vi "NI.Relays.vi"(6 "测试日志信息":refnum<queue>, 8 "error in":errorcluster caption="Error In", 9 "Relay.ON.OFF":bool caption="Relay.ON/OFF", 10 "Relay":T1(ring), 11 "DAQmx Device":tag) -> (0 "error out":errorcluster caption="Error Out")   [LabVIEW 2012, in "Lib_UEL.ATE.lvlib" / "Lib_PCI6221.lvlib"]
uses:
  Lib_PCI6221.lvlib
  <vilib>/DAQmx/write.llb/DAQmx Write (Digital Bool 1Line 1Point).vi
  <vilib>/DAQmx/create/channels.llb/DAQmx Create Channel (DO-Digital Output).vi
  <vilib>/DAQmx/miscellaneous.llb/DAQmx Fill In Error Info.vi
panel:
  # "V01 - Initial version. ~LiGuang 2011-05-12 \n V02 - 2013/1/11, 增加测试日志功能: 将测试信息加入到输入的队列中."
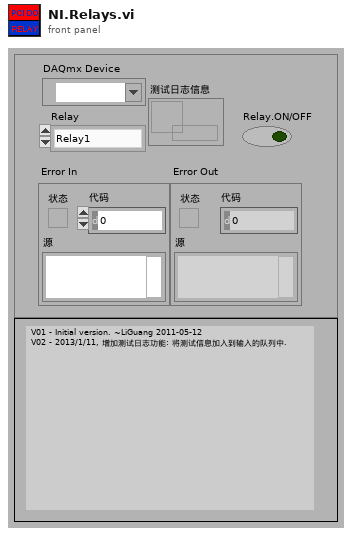
[diagram p1: front panel]
types:
  T1 = enum16{"Relay1", "Relay2", "Relay3", "Relay4", "Relay5", "Relay6", "Relay7", "Relay8", "Relay9", "Relay10"}
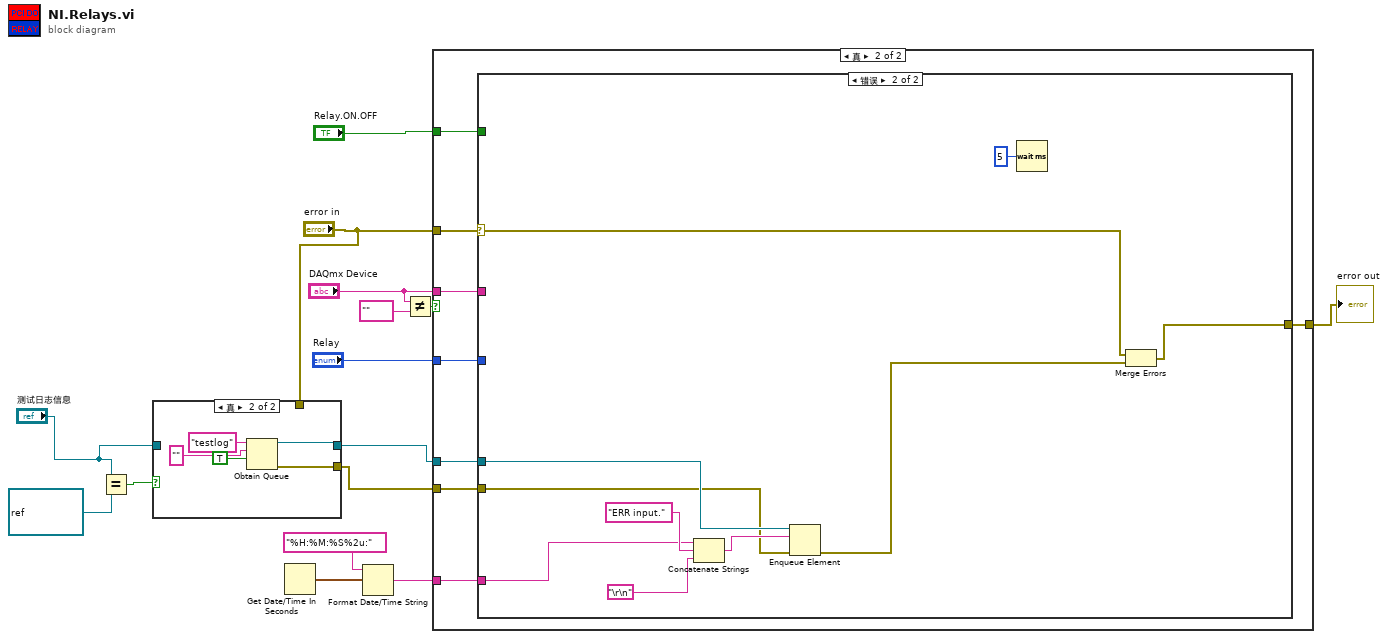
[diagram p0: block diagram]
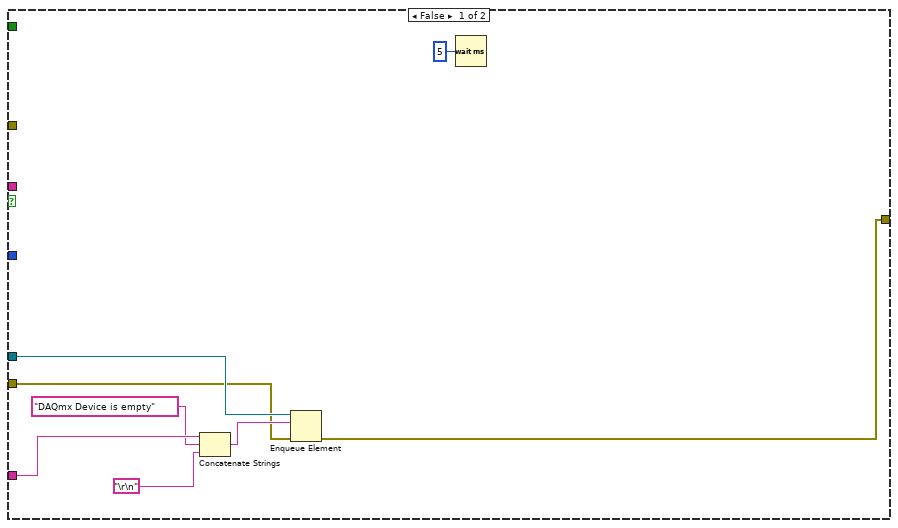
[diagram p3: hidden frame]
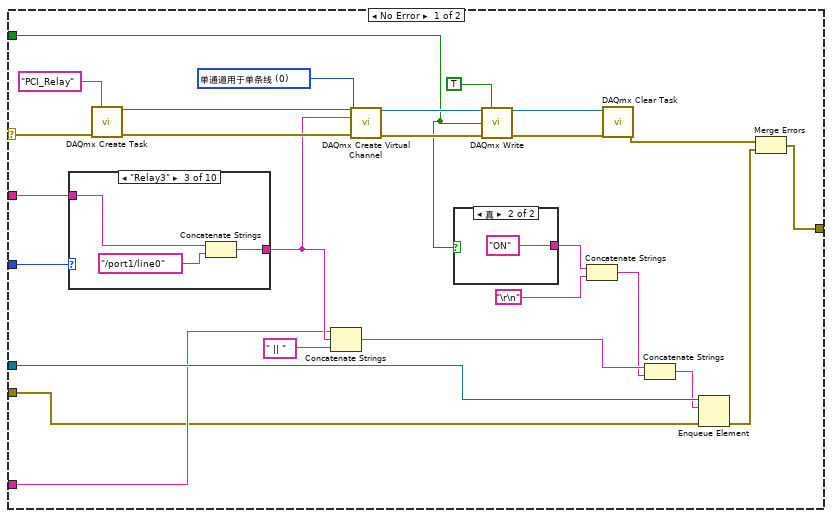
[diagram p4: hidden frame]
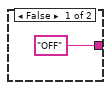
[diagram p5: hidden frame]
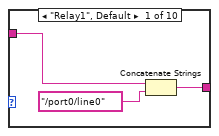
[diagram p6: hidden frame]
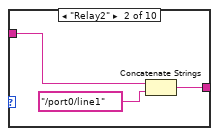
[diagram p7: hidden frame]
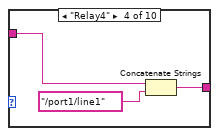
[diagram p8: hidden frame]
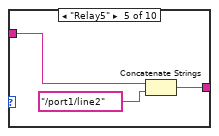
[diagram p9: hidden frame]
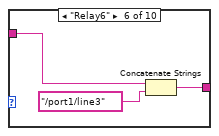
[diagram p10: hidden frame]
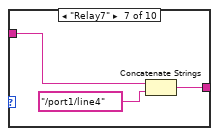
[diagram p11: hidden frame]
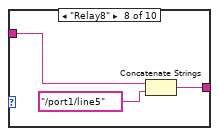
[diagram p12: hidden frame]
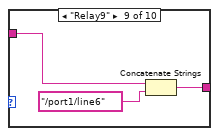
[diagram p13: hidden frame]
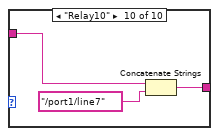
[diagram p14: hidden frame]
diagram:
  n1 = Equal?(x="测试日志信息", y=refnum<queue> refnum) -> (x = y?=w5:bool)
  n2 = case shown="真" w5 {
    tunnel: "测试日志信息" -> [w17 _]
    tunnel: [w17 w22] -> w3
    tunnel: [w16 w21] -> w1
    tunnel: "error in" -> [w16 _]
    frame False {
    }
    frame True {
      n3 = Obtain Queue(name (unnamed)="testlog" ("名称（未命名）"), element data type="" ("名称（未命名）"), create if not found? (T)=TRUE ("如未找到是否创建？(T)")) -> (queue out=w22:refnum<queue>, error out=w21:errorcluster)  [unwired: 2 in, 1 out]
    }
  }
  n4 = Get Date/Time In Seconds() -> (seconds since 1Jan1904=w8:timestamp)
  n5 = Format Date/Time String(time format string (%c)="%H:%M:%S%2u:" ("时间格式化字符串(%c)"), seconds (now)=w8) -> (date/time string=w7:string)  [unwired: 1 in]
  n6 = Not Equal?(x="DAQmx Device", y=tag "") -> (x != y?=w10:bool)
  n7 = case shown="真" w10 {
    tunnel: "error in" -> [_ w38]
    tunnel: [w25 w37] -> w15
    tunnel: "Relay" -> [_ w36]
    tunnel: "Relay.ON.OFF" -> [_ w35]
    tunnel: "DAQmx Device" -> [_ w34]
    tunnel: w3 -> [w30 w33]
    tunnel: w7 -> [w29 w32]
    tunnel: w1 -> [w23 w31]
    frame False {
      n8 = Concatenate Strings(w29, "DAQmx Device is empty" ("时间格式化字符串(%c)"), "\r\n") -> (w26:string)
      n9 = Enqueue Element(queue=w30, element=w26, error in (no error)=w23) -> (error out=w25:errorcluster)  [unwired: 1 in, 2 out]
      n10 = Wait (ms)(milliseconds to wait=u32 5 ("等待时间（毫秒）")) -> ()  [unwired: 1 out]
    }
    frame True {
      n11 = case shown="错误" w38 {
        selector: w38 -> [w52 w101]
        tunnel: [w49 w104] -> w37
        tunnel: w36 -> [w61 _]
        tunnel: w34 -> [w60 _]
        tunnel: w35 -> [w45 _]
        tunnel: w33 -> [w53 w106]
        tunnel: w32 -> [w47 w100]
        tunnel: w31 -> [w39 w97]
        frame No Error {
          w59 = 0 items=["单通道用于单条线", "单通道用于所有线"] ("line grouping")
          n12 = case shown="\"Relay3\"" w61 {
            tunnel: w60 -> [w68 w71 w74 w77 w80 w83 w86 w89 w92 w95]
            tunnel: [w67 w70 w73 w76 w79 w82 w85 w88 w91 w94] -> w48
            frame "Relay1", Default {
              n13 = Concatenate Strings(w68, "/port0/line0") -> (w67:string)
            }
            frame "Relay2" {
              n14 = Concatenate Strings(w71, "/port0/line1") -> (w70:string)
            }
            frame "Relay3" {
              n15 = Concatenate Strings(w74, "/port1/line0") -> (w73:string)
            }
            frame "Relay4" {
              n16 = Concatenate Strings(w77, "/port1/line1") -> (w76:string)
            }
            frame "Relay5" {
              n17 = Concatenate Strings(w80, "/port1/line2") -> (w79:string)
            }
            frame "Relay6" {
              n18 = Concatenate Strings(w83, "/port1/line3") -> (w82:string)
            }
            frame "Relay7" {
              n19 = Concatenate Strings(w86, "/port1/line4") -> (w85:string)
            }
            frame "Relay8" {
              n20 = Concatenate Strings(w89, "/port1/line5") -> (w88:string)
            }
            frame "Relay9" {
              n21 = Concatenate Strings(w92, "/port1/line6") -> (w91:string)
            }
            frame "Relay10" {
              n22 = Concatenate Strings(w95, "/port1/line7") -> (w94:string)
            }
          }
          n23 = call <vilib>:"DAQmx Create Task.vi"("new task name"="PCI_Relay", "error in"=w52) -> ("task out"=w62:refnum<k21>, "error out"=w63:errorcluster)  [unwired: 12 in]
          n24 = Concatenate Strings(w47, w48, " || ") -> (w42:string)
          n25 = call-poly <vilib>:"DAQmx Create Virtual Channel.vi"("task in"=w62, "lines"=w48, "line grouping"=w59, "error in"=w63) -> ("task out"=w58:refnum<k21>, "error out"=w57:errorcluster)  [unwired: 10 in]
          n26 = case shown="真" w45 {
            tunnel: ["OFF" "ON"] -> w44
            frame False {
            }
            frame True {
            }
          }
          n27 = call-poly <vilib>:"DAQmx Write.vi"("task/channels in"=w58, "auto start"=TRUE, "data"=w45, "error in"=w57) -> ("task out"=w55:refnum<k21>, "error out"=w54:errorcluster)  [unwired: 9 in, 1 out]
          n28 = Concatenate Strings(w44, "\r\n") -> (w41:string)
          n29 = call <vilib>:"DAQmx Clear Task.vi"("task in"=w55, "error in"=w54) -> ("error out"=w51:errorcluster)  [unwired: 13 in]
          n30 = Concatenate Strings(w42, w41) -> (w40:string)
          n31 = Enqueue Element(queue=w53, element=w40, error in (no error)=w39) -> (error out=w50:errorcluster)  [unwired: 1 in, 2 out]
          n32 = Merge Errors(w51, w50) -> (w49:errorcluster)
        }
        frame Error {
          n33 = Concatenate Strings(w100, "ERR input." ("时间格式化字符串(%c)"), "\r\n") -> (w99:string)
          n34 = Enqueue Element(queue=w106, element=w99, error in (no error)=w97) -> (error out=w105:errorcluster)  [unwired: 1 in, 2 out]
          n35 = Wait (ms)(milliseconds to wait=u32 5 ("等待时间（毫秒）")) -> ()  [unwired: 1 out]
          n36 = Merge Errors(w101, w105) -> (w104:errorcluster)
        }
      }
    }
  }
  "error out" <- w15
